vi "4_Osciloscopio.vi"() -> ()   [LabVIEW 2020]
panel:
  in  "stop":bool
  out "Waveform Chart":dynamicdata(graph)
  in  "Phase":dbl
  in  "Frequency":dbl=10.1
  in  "Amplitude":dbl=1.0
  in  "Reset Signal":bool
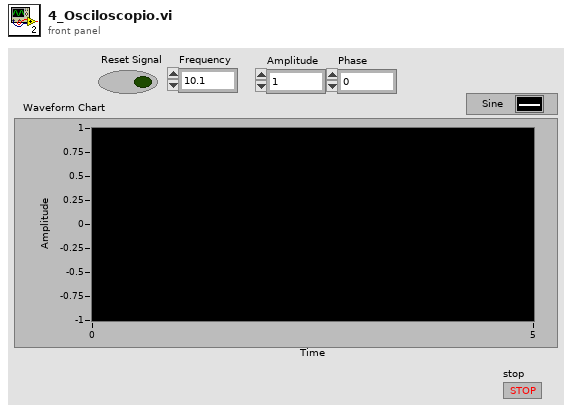
[diagram p1: front panel]
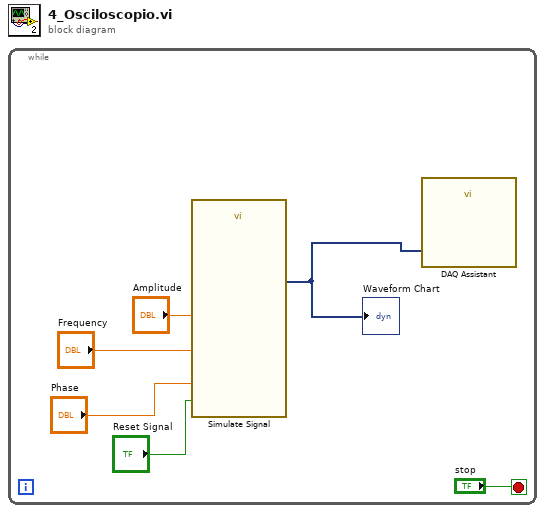
[diagram p0: block diagram]
diagram:
  n1 = while {
    stop <- "stop" stop-if-true
    n2 = call "Simulate Signal"("Reset Signal"="Reset Signal", "Frequency"="Frequency", "Amplitude"="Amplitude", "Phase"="Phase") -> ("Sine"=w1:dynamicdata)  [unwired: 10 in, 1 out]
    "Waveform Chart" <- w1
    n3 = call "DAQ Assistant"("data"=w1) -> ()  [unwired: 17 in, 2 out]
  }
